vi "Reset.vi"(8 "error in (no error)":errorcluster, 11 "VISA resource name":refnum<visa-resource-name>) -> (0 "error out":errorcluster, 3 "VISA resource name out":refnum<visa-resource-name>)   [LabVIEW 2018, in "JULABO DeviceDriver.lvlib"]
doc: "Resets the instrument and then sends a set of default setup commands to the instrument."
uses:
  JULABO DeviceDriver.lvlib
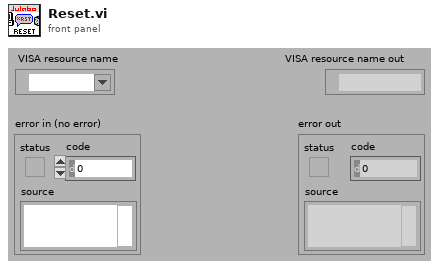
[diagram p1: front panel]
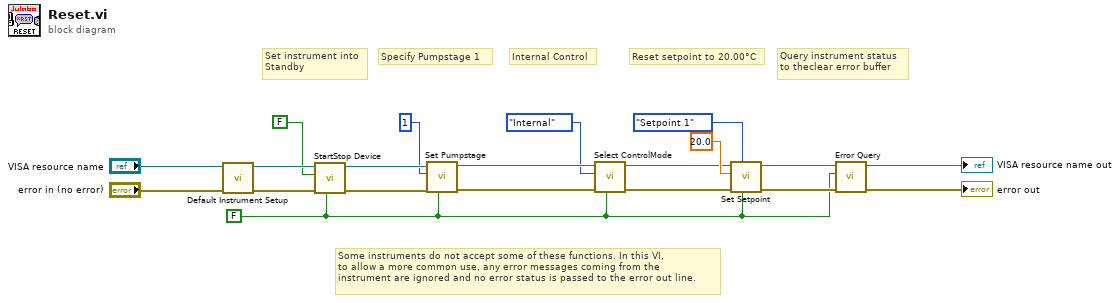
[diagram p0: block diagram]
diagram:
  w1 = FALSE ("parseError? T:Yes")
  # "Some instruments do not accept some of these functions. In this VI,\nto allow a more common use, any error messages coming from the\ninstrument are ignored and no error status is passed to the error out line."
  # "Query instrument status\nto theclear error buffer"
  # "Reset setpoint to 20.00°C"
  # "Internal Control"
  # "Specify Pumpstage 1"
  # "Set instrument into\nStandby"
  n1 = call "Default Instrument Setup.vi"("error in (no error)"="error in (no error)", "VISA resource name"="VISA resource name") -> ("error out"=w20:errorcluster, "VISA resource name out"=w19:refnum<visa-resource-name>)  [unwired: 8 in]
  n2 = call "StartStop Device.vi"("parseError? T:Yes"=w1, "error in (no error)"=w20, "Start/Stop (f:Stop)"=FALSE, "VISA resource name"=w19) -> ("error out"=w17:errorcluster, "VISA resource name out"=w18:refnum<visa-resource-name>)  [unwired: 6 in]
  n3 = call "Set Pumpstage.vi"("parseError? T:Yes"=w1, "error in (no error)"=w17, "Pumpstage (1: default)"=u8 1, "VISA resource name"=w18) -> ("error out"=w13:errorcluster, "VISA resource name out"=w14:refnum<visa-resource-name>)  [unwired: 6 in]
  n4 = call "Select ControlMode.vi"("parseError? T:Yes"=w1, "error in (no error)"=w13, "Control (0: Internal)"=enum16{"Internal", "External"}."Internal", "VISA resource name"=w14) -> ("error out"=w11:errorcluster, "VISA resource name out"=w12:refnum<visa-resource-name>)  [unwired: 6 in]
  n5 = call "Set Setpoint.vi"("parseError? T:Yes"=w1, "Setpointindex (Setpoint1: Default)"=enum16{"Setpoint 1", "Setpoint 2", "Setpoint 3"}."Setpoint 1" ("Setpoint (Setpoint1: Default)"), "error in (no error)"=w11, "newSetpoint (20.00°C)"=20.0, "VISA resource name"=w12) -> ("error out"=w4:errorcluster, "VISA resource name out"=w5:refnum<visa-resource-name>)  [unwired: 5 in]
  n6 = call "Error Query.vi"("error in (no error)"=w4, "parseError? (true)"=w1, "VISA resource name"=w5) -> ("error out"=→"error out":errorcluster, "VISA resource name out"=→"VISA resource name out":refnum<visa-resource-name>)  [unwired: 5 in, 2 out]
